vi "XtoY.vi"(1 "X":i32, 2 "Y":i32) -> (0 "Result":T1)   [LabVIEW 2025]
uses:
  Number.ctl
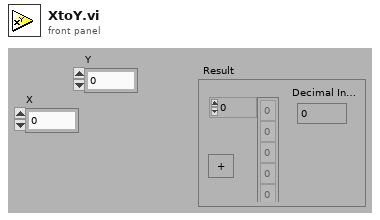
[diagram p1: front panel]
types:
  T1 = typedef "Number.ctl" = cluster{"Array Num":i8[], "Decimal Index":i32, "stop":bool}
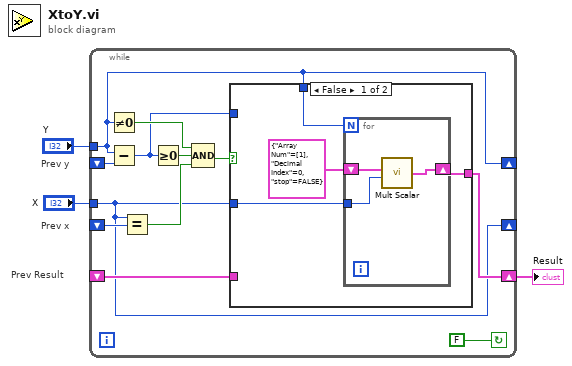
[diagram p0: block diagram]
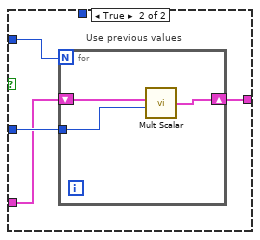
[diagram p2: hidden frame]
diagram:
  # "Prev Result"
  # "Prev y"
  # "Prev x"
  n1 = while {
    tunnel: "X" -> [w6]
    shift-right: [w6] -> _
    shift-left: _ -> [w15]
    tunnel: "Y" -> [w5]
    shift-right: [w5] -> _
    shift-left: _ -> [w12]
    shift-right: [w7] -> w1
    shift-left: _ -> [w8]
    stop <- FALSE continue-if-true
    n2 = Not Equal To 0?(x=w5) -> (x != 0?=w10:bool)
    n3 = Subtract(x=w5, y=w12) -> (x-y=w9:i32)
    n4 = Equal?(x=w6, y=w15) -> (x = y?=w14:bool)
    n5 = Greater Or Equal To 0?(x=w9) -> (x >= 0?=w11:bool)
    n6 = Compound Arithmetic op=AND(w10, w11, w14) -> (w13:bool)
    n7 = case shown="False" w13 {
      tunnel: w6 -> [w18 w26]
      tunnel: [w16 w23] -> w7
      tunnel: w9 -> [_ w25]
      tunnel: w8 -> [_ w24]
      tunnel: w5 -> [w19 _]
      frame False {
        n8 = for {
          N: w19 -> [_]
          tunnel: w18 -> [w22]
          shift-right: [w20] -> w16
          shift-left: T1 {"Array Num"=[1], "Decimal Index"=0, "stop"=FALSE} ("A x Scalar") -> [w21]
          n9 = call "Mult Scalar.vi"("A"=w21, "Scalar"=w22) -> ("A x Scalar"=w20:T1)  [unwired: 3 in]
        }
      }
      frame True {
        # "Use previous values"
        n10 = for {
          N: w25 -> [_]
          tunnel: w26 -> [w27]
          shift-right: [w28] -> w23
          shift-left: w24 -> [w29]
          n11 = call "Mult Scalar.vi"("A"=w29, "Scalar"=w27) -> ("A x Scalar"=w28:T1)  [unwired: 3 in]
        }
      }
    }
  }
  "Result" <- w1
